vi "DLL Retcode to VI Errcode.vi"(8 "error in (no error)":errorcluster, 11 "DLL Retcode":i32 format="%x") -> (0 "error out":errorcluster, 3 "VI Errcode":i32 format="%x")   [LabVIEW 2024, in "Keyence LK-G3000.lvlib"]
uses:
  Keyence LK-G3000.lvlib
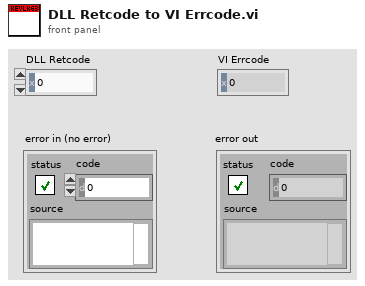
[diagram p1: front panel]
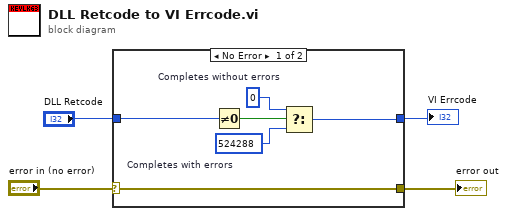
[diagram p0: block diagram]
diagram:
  n1 = case shown="No Error" "error in (no error)" {
    selector: "error in (no error)" -> [w10 w11]
    tunnel: [w10 w11] -> w3
    tunnel: "DLL Retcode" -> [w7 w12]
    tunnel: [w9 w12] -> w1
    frame No Error {
      w5 = 524288  # Completes with errors
      w6 = 0  # Completes without errors
      n2 = Not Equal To 0?(x=w7) -> (x != 0?=w8:bool)
      n3 = Select(t=w6, s=w8, f=w5) -> (s? t:f=w9:i32)
    }
    frame Error {
    }
  }
  "error out" <- w3
  "VI Errcode" <- w1
